vi "Write test data to sql database polaris.vi"(6 "error in (no error)":errorcluster, 9 "Serial":string) -> (0 "error out":errorcluster, 1 "No dup serial?":bool, 2 "Test rec csv line":string, 3 "Passed?":bool)   [LabVIEW 2013]
uses:
  Test Globals/Global 1.vi
  Main Support/Global 2.vi
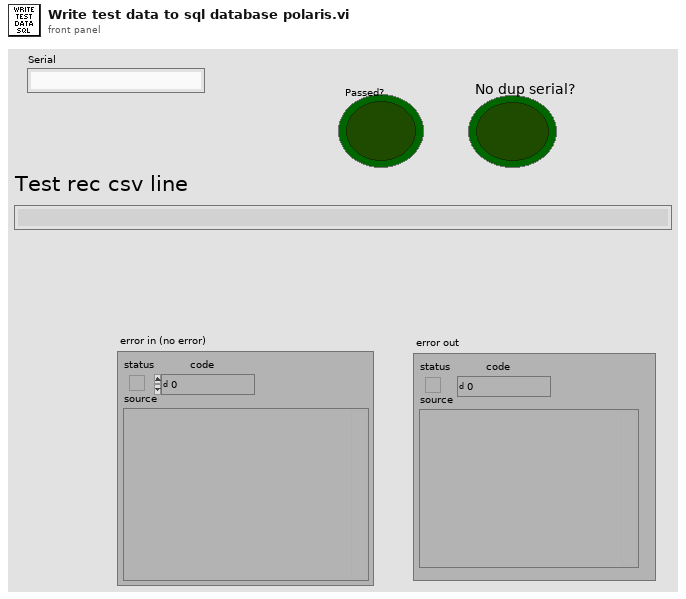
[diagram p1: front panel]
types:
  T1 = enum16{"Query", "Insert", "Select", "Dump Recs", "Get Rec Count", "Get Col Names", "Insert all fields", "Find", "Get last test result", "Get work order qty", "Set work order qty", "Save test report", "Get test report", "Execute query no data", "Select count", "Query and return row 0 col 0"}
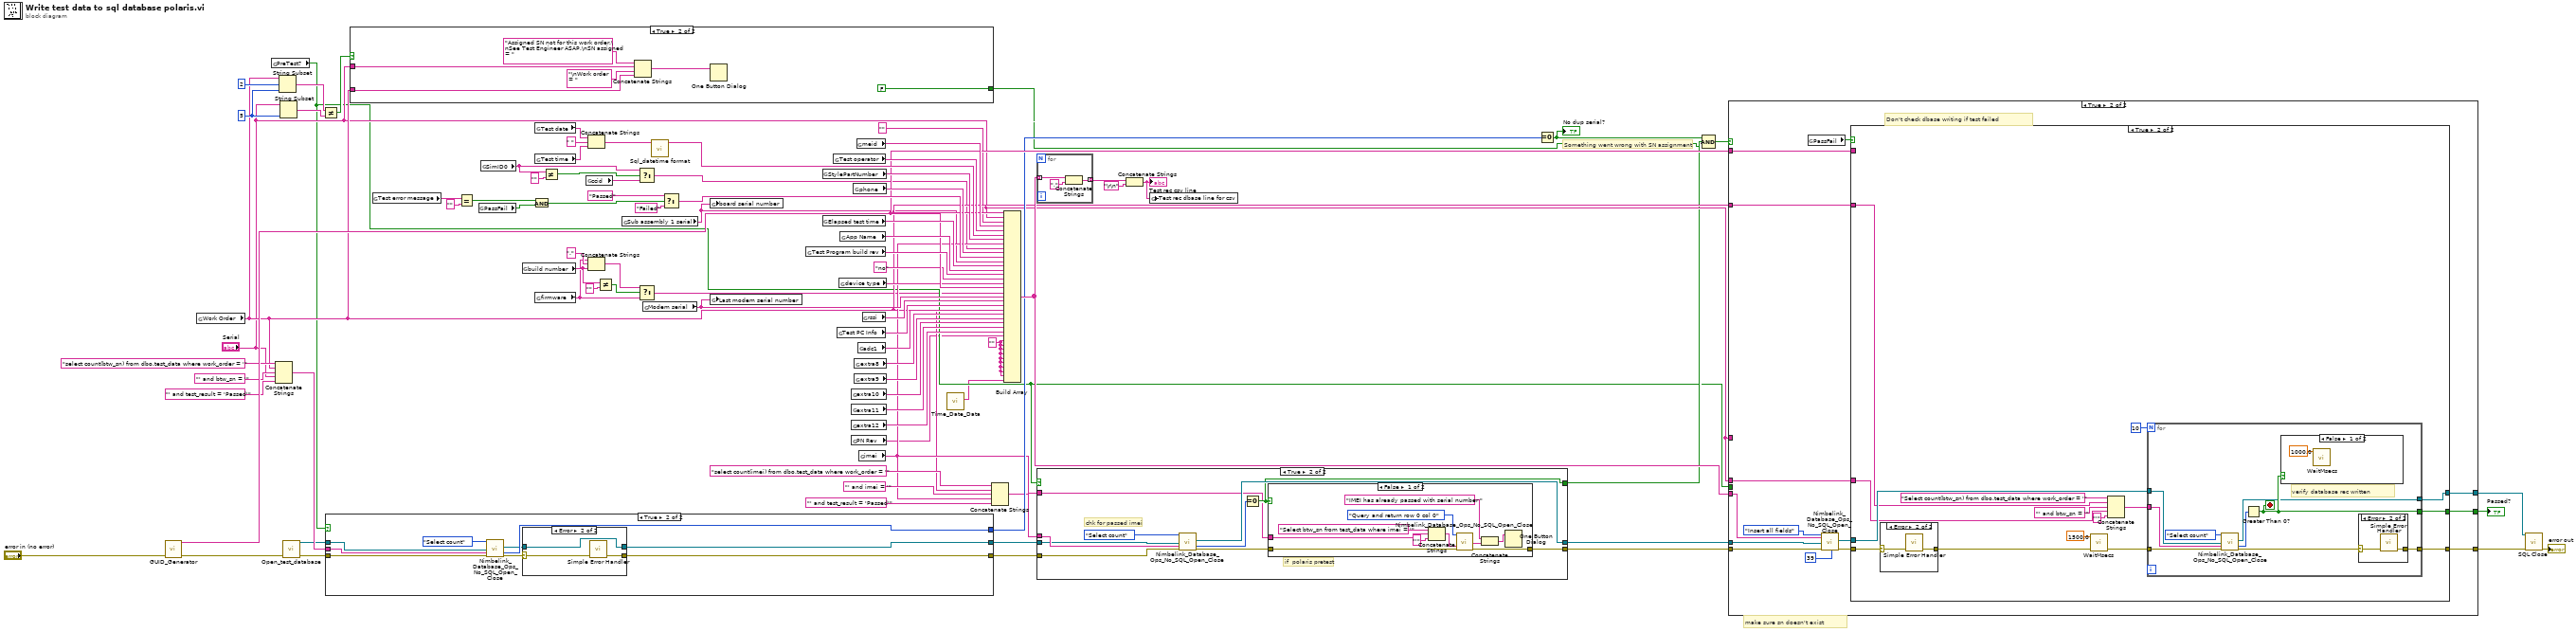
[diagram p0: block diagram]
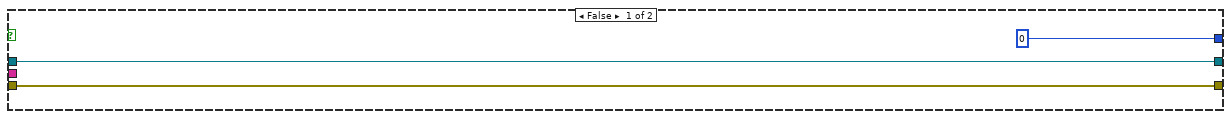
[diagram p2: hidden frame]
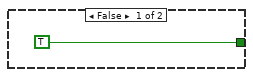
[diagram p4: hidden frame]
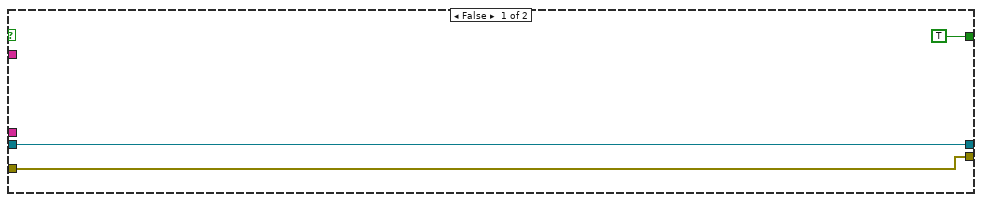
[diagram p5: hidden frame]
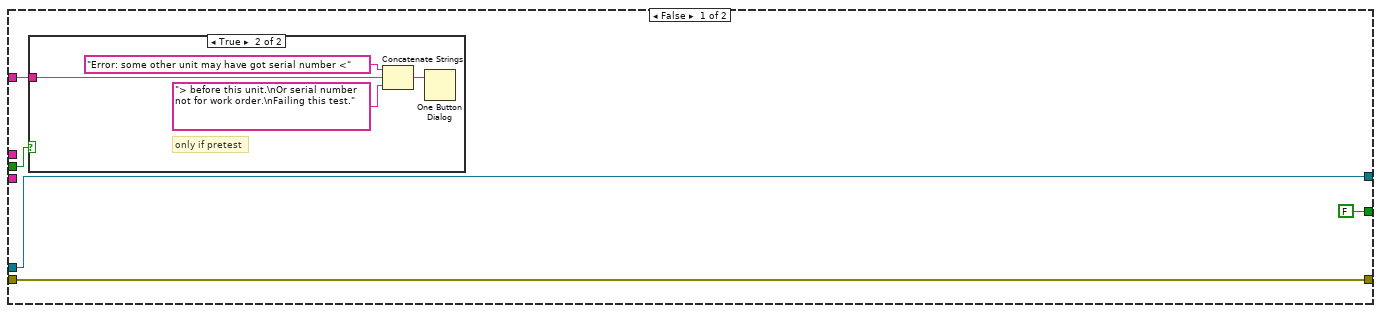
[diagram p7: hidden frame]
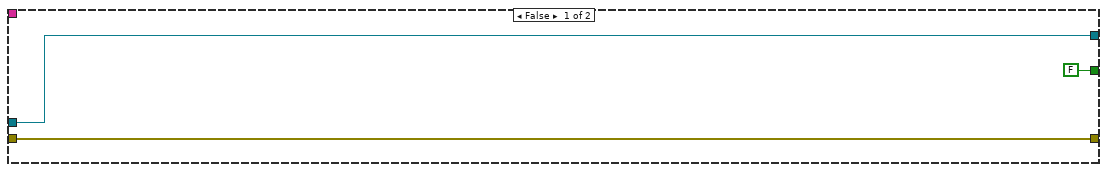
[diagram p9: hidden frame]
diagram:
  w15 = "" ("element")
  w29 = 5 ("length (rest)")
  # "Something went wrong with SN assignment"
  # "make sure sn doesn't exist"
  n1 = call "GUID_Generator.vi"("error in (no error)"="error in (no error)") -> ("error out"=w63:errorcluster, "GUID String"=w66:string)  [unwired: 9 in]
  n2 = global read "Global 2.vi" "Work Order"() -> (w25:string)
  n3 = global read "Global 1.vi" "PreTest?"() -> (w16:bool)
  n4 = Concatenate Strings("select count(btw_sn) from dbo.test_data where work_order = '" ("SQL Query"), w25, "' and btw_sn = '" ("string"), "Serial", "' and test_result = 'Passed'" ("string")) -> (w48:string)
  n5 = String Subset(string=w25, offset (0)=2, length (rest)=w29) -> (substring=w28:string)
  n6 = String Subset(string="Serial", length (rest)=w29) -> (substring=w27:string)  [unwired: 1 in]
  n7 = call "Open_test_database.vi"("error in (no error)"=w63) -> ("error out"=w52:errorcluster, "SQL conn Refnum out"=w46:refnum<k7>)  [unwired: 9 in]
  n8 = Not Equal?(x=w28, y=w27) -> (x != y?=w26:bool)
  n9 = case shown="True" w16 {
    tunnel: w52 -> [w89 w99]
    tunnel: w48 -> [_ w97]
    tunnel: [0 ("Records") w96] -> w47
    tunnel: w46 -> [w88 w95]
    tunnel: [w89 w93] -> w41
    tunnel: [w88 w91] -> w39
    frame False {
    }
    frame True {
      n10 = call "Nimbelink_Database_Ops_No_SQL_Open_Close.vi"("Operation"=T1."Select count", "Connection In"=w95, "SQL Query"=w97, "Error in (no error)"=w99) -> ("Connection Out"=w92:refnum<k7>, "Records"=w96:i32, "Error out"=w94:errorcluster)  [unwired: 8 in, 5 out]
      n11 = case shown="Error" w94 {
        selector: w94 -> [w101 w104]
        tunnel: [w101 w103] -> w93
        tunnel: w92 -> [w100 w102]
        tunnel: [w100 w102] -> w91
        frame No Error {
        }
        frame Error {
          n12 = call <vilib>:"Simple Error Handler.vi"("error in (no error)"=w104) -> ("error out"=w103:errorcluster)  [unwired: 4 in, 4 out]
        }
      }
    }
  }
  n13 = case shown="True" w26 {
    tunnel: "Serial" -> [_ w109]
    tunnel: w25 -> [_ w107]
    tunnel: [TRUE FALSE] -> w21
    frame False {
    }
    frame True {
      n14 = Concatenate Strings("Assigned SN not for this work order.\nSee Test Engineer ASAP.\nSN assigned = " ("string"), w109, "\nWork order = " ("string"), w107) -> (w111:string)
      n15 = One Button Dialog(message=w111) -> ()  [unwired: 1 in, 1 out]
    }
  }
  n16 = global read "Global 1.vi" "Test error message"() -> (w72:string)
  n17 = Equal?(x=w72, y="") -> (x = y?=w70:bool)
  n18 = global read "Global 2.vi" "PassFail"() -> (w68:bool)
  n19 = global read "Global 1.vi" "SimID0"() -> (w11:string)
  n20 = global read "Global 1.vi" "build number"() -> (w7:string)
  n21 = And(x=w70, y=w68) -> (x .and. y?=w67:bool)
  n22 = global read "Global 2.vi" "Test date"() -> (w86:string)
  n23 = global read "Global 2.vi" "Test time"() -> (w84:string)
  n24 = global read "Global 1.vi" "firmware"() -> (w3:string)
  n25 = Not Equal?(x=w11, y="") -> (x != y?=w12:bool)
  n26 = global read "Global 1.vi" "ccid"() -> (w10:string)
  n27 = Concatenate Strings(w86, " " ("string"), w84) -> (w79:string)
  n28 = Concatenate Strings(w3, "." ("string"), w7) -> (w4:string)
  n29 = Not Equal?(x=w7, y="") -> (x != y?=w5:bool)
  n30 = global read "Global 1.vi" "Sub assembly 1 serial"() -> (w17:string)
  n31 = Select(t=w11, s=w12, f=w10) -> (s? t:f=w9:string)
  n32 = Select(t=w4, s=w5, f=w3) -> (s? t:f=w2:string)
  n33 = global read "Global 1.vi" "Modem serial"() -> (w32:string)
  n34 = call "Sql_datetime format.vi"("Date time In"=w79) -> ("Sql datetime type 20"=w78:string)  [unwired: 9 in, 1 out]
  n35 = Select(t="Passed" ("element"), s=w67, f="Failed" ("element")) -> (s? t:f=w73:string)
  n36 = global write "Global 1.vi" "board serial number"(w17) -> ()
  n37 = global write "Global 2.vi" "Last modem serial number"(w32) -> ()
  n38 = global read "Global 2.vi" "Test Program build rev"() -> (w75:string)
  n39 = global read "Global 2.vi" "StylePartNumber"() -> (w81:string)
  n40 = global read "Global 2.vi" "Elapsed test time"() -> (w77:string)
  n41 = global read "Global 2.vi" "Test operator"() -> (w82:string)
  n42 = global read "Global 2.vi" "Test PC Info"() -> (w59:string)
  n43 = global read "Global 1.vi" "device type"() -> (w65:string)
  n44 = global read "Global 2.vi" "App Name"() -> (w76:string)
  n45 = global read "Global 1.vi" "extra10"() -> (w35:string)
  n46 = global read "Global 1.vi" "extra11"() -> (w34:string)
  n47 = global read "Global 1.vi" "extra12"() -> (w33:string)
  n48 = global read "Global 2.vi" "PN Rev"() -> (w14:string)
  n49 = global read "Global 1.vi" "phone"() -> (w80:string)
  n50 = global read "Global 1.vi" "extra8"() -> (w37:string)
  n51 = global read "Global 1.vi" "extra9"() -> (w36:string)
  n52 = global read "Global 1.vi" "meid"() -> (w83:string)
  n53 = global read "Global 1.vi" "adc1"() -> (w57:string)
  n54 = global read "Global 1.vi" "imei"() -> (w31:string)
  n55 = global read "Global 1.vi" "rssi"() -> (w60:string)
  n56 = call "Time_Date_Data.vi"() -> ("UTC ISO 8601"=w1:string)  [unwired: 4 in, 7 out]
  n57 = Concatenate Strings("select count(imei) from dbo.test_data where work_order = '" ("SQL Query"), w25, "' and imei = '" ("string"), w31, "' and test_result = 'Passed'" ("string")) -> (w42:string)
  n58 = Build Array(w25, "Serial", "" ("element"), w83, w82, w78, w81, w31, w9, w80, w73, w17, w77, w76, w75, "no" ("element"), w65, w66, w2, w32, w60, w59, w57, w37, w36, w35, w34, w33, w14, w15, w15, w15, w15, w15, w15, w15, w15, w15, w1) -> (w56:string[])
  n59 = for {
    tunnel: w56 -> [w114] mode=indexing
    tunnel: [w112] -> w55 mode=indexing
    n60 = Concatenate Strings(w114, "," ("string")) -> (w112:string)
  }
  n61 = case shown="True" w16 {
    tunnel: w42 -> [_ w126]
    tunnel: [TRUE w121] -> w22
    tunnel: w41 -> [w116 w124]
    tunnel: [w116 w119] -> w40
    tunnel: w39 -> [w115 w123]
    tunnel: [w115 w122] -> w38
    tunnel: w31 -> [_ w118]
    frame False {
    }
    frame True {
      # "if  polaris pretest"
      # "chk for passed imei"
      n62 = call "Nimbelink_Database_Ops_No_SQL_Open_Close.vi"("Operation"=T1."Select count", "Connection In"=w123, "SQL Query"=w126, "Error in (no error)"=w124) -> ("Connection Out"=w122:refnum<k7>, "Records"=w125:i32, "Error out"=w120:errorcluster)  [unwired: 8 in, 5 out]
      n63 = Equal To 0?(x=w125) -> (x = 0?=w121:bool)
      n64 = case shown="False" w121 {
        tunnel: w120 -> [w137 w138]
        tunnel: [w136 w138] -> w119
        tunnel: w118 -> [w133 _]
        frame False {
          n65 = Concatenate Strings("Select btw_sn from test_data where imei = '" ("SQL Query"), w133, "'" ("string")) -> (w131:string)
          n66 = call "Nimbelink_Database_Ops_No_SQL_Open_Close.vi"("Operation"=T1."Query and return row 0 col 0", "SQL Query"=w131, "Error in (no error)"=w137) -> ("Find return string"=w129:string, "Error out"=w136:errorcluster)  [unwired: 9 in, 6 out]
          n67 = Concatenate Strings("IMEI has already passed with serial number " ("message"), w129) -> (w128:string)
          n68 = One Button Dialog(message=w128) -> ()  [unwired: 1 in, 1 out]
        }
        frame True {
        }
      }
    }
  }
  n69 = Concatenate Strings(w55, "\r\n") -> (w53:string)
  "Test rec csv line" <- w53
  n70 = global write "Global 1.vi" "Test rec dbase line for csv"(w53) -> ()
  n71 = Equal To 0?(x=w47) -> (x = 0?=w23:bool)
  "No dup serial?" <- w23
  n72 = Compound Arithmetic op=AND(w23, w22, w21) -> (w20:bool)
  n73 = case shown="True" w20 {
    tunnel: [FALSE w161] -> w19
    tunnel: w66 -> [_ w160]
    tunnel: w38 -> [w142 w159]
    tunnel: [w143 w158] -> w62
    tunnel: [w142 w157] -> w61
    tunnel: w56 -> [_ w156]
    tunnel: w25 -> [_ w155]
    tunnel: "Serial" -> [_ w154]
    tunnel: w40 -> [w143 w153]
    tunnel: "Serial" -> [w140 _]
    tunnel: w16 -> [w139 _]
    frame False {
      n74 = case shown="True" w139 {
        tunnel: w140 -> [_ w146]
        frame False {
        }
        frame True {
          # "only if pretest"
          n75 = Concatenate Strings("Error: some other unit may have got serial number <" ("message"), w146, "> before this unit.\nOr serial number not for work order.\nFailing this test." ("string")) -> (w144:string)
          n76 = One Button Dialog(message=w144) -> ()  [unwired: 1 in, 1 out]
        }
      }
    }
    frame True {
      # "Don't check dbase writing if test failed"
      n77 = global read "Global 2.vi" "PassFail"() -> (w149:bool)
      n78 = call "Nimbelink_Database_Ops_No_SQL_Open_Close.vi"("Operation"=T1."Insert all fields", "Record data"=w156, "Connection In"=w159, "Error in (no error)"=w153, "Insert fields"=39) -> ("Connection Out"=w150:refnum<k7>, "Error out"=w151:errorcluster)  [unwired: 7 in, 6 out]
      n79 = case shown="True" w149 {
        tunnel: w160 -> [_ _]
        tunnel: [FALSE w176] -> w161
        tunnel: [w164 w175] -> w158
        tunnel: w151 -> [w164 w166]
        tunnel: w150 -> [w163 w171]
        tunnel: [w163 w170] -> w157
        tunnel: w155 -> [_ w169]
        tunnel: w154 -> [_ w168]
        frame False {
        }
        frame True {
          n80 = case shown="Error" w166 {
            selector: w166 -> [w180 w182]
            tunnel: [w180 w181] -> w165
            frame No Error {
            }
            frame Error {
              n81 = call <vilib>:"Simple Error Handler.vi"("error in (no error)"=w182) -> ("error out"=w181:errorcluster)  [unwired: 4 in, 4 out]
            }
          }
          n82 = call "WaitMsecs.vi"("error in (no error)"=w165, "Wait Msecs"=1500.0) -> ("error out"=w172:errorcluster)  [unwired: 9 in]
          n83 = Concatenate Strings("Select count(btw_sn) from dbo.test_data where work_order = '" ("SQL Query"), w169, "' and btw_sn = '" ("string"), w168, "'" ("string")) -> (w177:string)
          n84 = for {
            N: 10 -> [_]
            tunnel: w177 -> [w191]
            tunnel: [w190] -> w176
            tunnel: [w183] -> w175
            tunnel: w172 -> [w189]
            tunnel: w171 -> [w186]
            tunnel: [w185] -> w170
            stop <- w190 stop-if-true
            # "verify database rec written"
            n85 = call "Nimbelink_Database_Ops_No_SQL_Open_Close.vi"("Operation"=T1."Select count", "Connection In"=w186, "SQL Query"=w191, "Error in (no error)"=w189) -> ("Connection Out"=w185:refnum<k7>, "Records"=w187:i32, "Error out"=w184:errorcluster)  [unwired: 8 in, 5 out]
            n86 = Greater Than 0?(x=w187) -> (x > 0?=w190:bool)
            n87 = case shown="False" w190 {
              frame False {
                n88 = call "WaitMsecs.vi"("Wait Msecs"=1000.0) -> ()  [unwired: 10 in, 1 out]
              }
              frame True {
              }
            }
            n89 = case shown="Error" w184 {
              selector: w184 -> [w192 w194]
              tunnel: [w192 w193] -> w183
              frame No Error {
              }
              frame Error {
                n90 = call <vilib>:"Simple Error Handler.vi"("error in (no error)"=w194) -> ("error out"=w193:errorcluster)  [unwired: 4 in, 4 out]
              }
            }
          }
        }
      }
    }
  }
  "Passed?" <- w19
  n91 = call "SQL Close.vi"("Connection In"=w61, "Error in (no error)"=w62) -> ("Error out"=→"error out":errorcluster)  [unwired: 17 in]
